vi "RAMP_close_single_scan_FPGA.vi"(0 "queue FPGA":refnum<queue>, 1 "queue ASI stage":refnum<queue>, 5 "queue CAMERA":refnum<queue>, 7 "Measure QPD":bool, 9 "queue piezo":refnum<queue>, 11 "error in":errorcluster, 12 "Z_position_file path":path, 14 "Illumination source":bool) -> (15 "error out":errorcluster)   [LabVIEW 2015]
uses:
  CONTROLS/Q_ASI_stage_element.ctl
  CONTROLS/Q_MCL_piezo_element.ctl
  CONTROLS/Q_camera_element.ctl
  CONTROLS/Q_FPGA_element.ctl
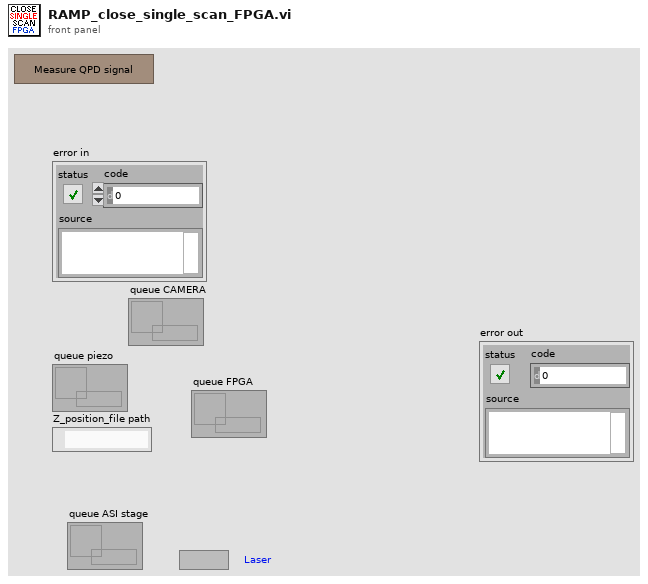
[diagram p1: front panel]
types:
  T1 = typedef "Q_FPGA_element.ctl" = cluster{"variant":variant, "Instruction":enum16{"FPGA_idle", "FPGA_initialize", "FPGA_error", "FPGA_security_stop", "FPGA_laser", "FPGA_start_stop_measure_QPD", "FPGA_measure_QPD", "FPGA_measure_QPD_noise", "FPGA_stop_measure_QPD", "FPGA_init_autofocus", "FPGA_init_single_scan", "FPGA_stop_single_scan", "FPGA_init_merFISH", "FPGA_measure_QPD_merFISH", "FPGA_init_scan_merFISH", "FPGA_scan_merFISH", "FPGA_close_merFISH", "FPGA_stop"}}
  T2 = typedef "Q_camera_element.ctl" = cluster{"variant":variant, "Instruction":enum16{"CAMERA_idle", "CAMERA_initialize", "CAMERA_error", "CAMERA_security_stop", "CAMERA_not_acquiring", "CAMERA_acquiring", "CAMERA_start_acquiring", "CAMERA_stop_acquiring", "CAMERA_change_exposure", "CAMERA_define_ROI", "CAMERA_cooler", "CAMERA_acquire_movie", "CAMERA_init_scan", "CAMERA_check_image_scan", "CAMERA_close_scan", "CAMERA_init_merFISH", "CAMERA_start_acquiring_merFISH", "CAMERA_close_scan_merFISH", "CAMERA_close_merFISH", "CAMERA_STOP"}}
  T3 = typedef "Q_MCL_piezo_element.ctl" = cluster{"variant":variant, "Instruction":enum16{"Piezo_idle", "Piezo_initialize", "Piezo_error", "Piezo_security_stop", "Piezo_read_z", "Piezo_move_z", "Piezo_keyboard_move", "Piezo_close_autofocus_calibration_ramp", "Piezo_change_init_state", "Piezo_init_autofocus", "Piezo_init_autofocus_merFISH_TL", "Piezo_autofocus", "Piezo_autofocus_merFISH_TL", "Piezo_stop_autofocus", "Piezo_stop_autofocus_merFISH_TL", "Piezo_autofocus_lost", "Piezo_resume_autofocus_merFISH_TL", "Piezo_check_z_position_merFISH_TL", "Piezo_init_ramp", "Piezo_move_z_ramp", "Piezo_close_ramp", "Piezo_close_merFISH", "Piezo_stop"}}
  T4 = typedef "Q_ASI_stage_element.ctl" = cluster{"variant":variant, "Instruction":enum16{"ASI_idle", "ASI_initialize", "ASI_error", "ASI_security_stop", "ASI_read_XYZ", "ASI_up", "ASI_down", "ASI_left", "ASI_right", "ASI_save_XY", "ASI_move_to_XY", "ASI_brightfield", "ASI_init_scan", "ASI_init_merFISH", "ASI_move_to_XY_merFISH", "ASI_move_to_Z_merFISH", "ASI_init_autofocus_search_merFISH", "ASI_close_autofocus_search_merFISH", "ASI_adjust_piezo_autofocus_merFISH", "ASI_set_piezo_autofocus_to_reference_position_merFISH_TL", "ASI_close_merFISH", "ASI_stop"}}
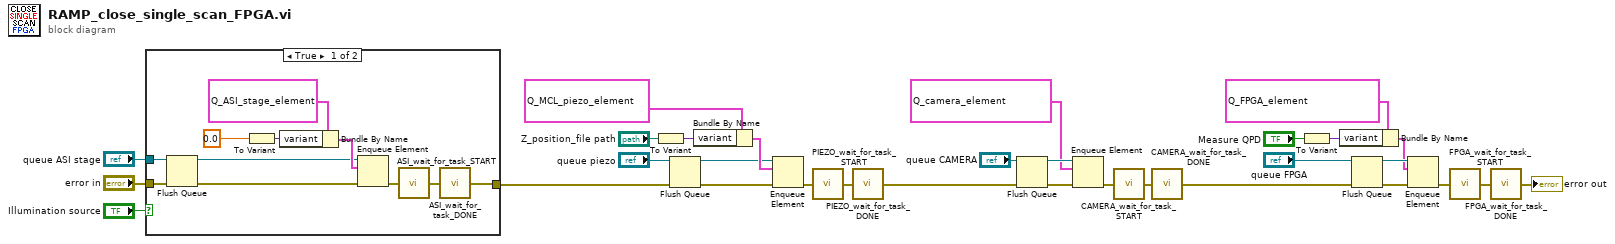
[diagram p0: block diagram]
diagram:
  n1 = case shown="True" "Illumination source" {
    tunnel: "error in" -> [w42 w43]
    tunnel: "queue ASI stage" -> [w41 _]
    tunnel: [w32 w43] -> w23
    frame True {
      n2 = Flush Queue(queue=w41, error in (no error)=w42) -> (queue out=w35:refnum<queue>, error out=w37:errorcluster)  [unwired: 1 out]
      n3 = To Variant(anything=0.0) -> (Variant=w39:variant)
      n4 = Bundle By Name(cluster=T4 {"variant"=variant, "Instruction"=enum."ASI_brightfield"} ("Q_ASI_stage"), "variant"=w39) -> (w36:T4)
      n5 = Enqueue Element(queue=w35, element=w36, error in (no error)=w37) -> (error out=w34:errorcluster)  [unwired: 1 in, 2 out]
      n6 = call "ASI_wait_for_task_START.vi"("error in"=w34) -> ("error out"=w33:errorcluster)
      n7 = call "ASI_wait_for_task_DONE.vi"("error in"=w33) -> ("error out"=w32:errorcluster)
    }
    frame False {
    }
  }
  n8 = To Variant(anything="Z_position_file path") -> (Variant=w22:variant)
  n9 = Flush Queue(queue="queue piezo", error in (no error)=w23) -> (queue out=w24:refnum<queue>, error out=w27:errorcluster)  [unwired: 1 out]
  n10 = Bundle By Name(cluster=T3 {"variant"=variant, "Instruction"=enum."Piezo_close_ramp"} ("Q_MCL_Piezo"), "variant"=w22) -> (w25:T3)
  n11 = Enqueue Element(queue=w24, element=w25, error in (no error)=w27) -> (error out=w20:errorcluster)  [unwired: 1 in, 2 out]
  n12 = call "PIEZO_wait_for_task_START.vi"("error in"=w20) -> ("error out"=w19:errorcluster)
  n13 = call "PIEZO_wait_for_task_DONE.vi"("error in"=w19) -> ("error out"=w14:errorcluster)
  n14 = Flush Queue(queue="queue CAMERA", error in (no error)=w14) -> (queue out=w16:refnum<queue>, error out=w15:errorcluster)  [unwired: 1 out]
  n15 = Enqueue Element(queue=w16, element=T2 {"variant"=variant, "Instruction"=enum."CAMERA_close_scan"} ("Q_ANDOR_element"), error in (no error)=w15) -> (error out=w17:errorcluster)  [unwired: 1 in, 2 out]
  n16 = call "CAMERA_wait_for_task_START.vi"("error in"=w17) -> ("error out"=w18:errorcluster)
  n17 = call "CAMERA_wait_for_task_DONE.vi"("error in"=w18) -> ("error out"=w11:errorcluster)
  n18 = To Variant(anything="Measure QPD") -> (Variant=w2:variant)
  n19 = Bundle By Name(cluster=T1 {"variant"=variant, "Instruction"=enum."FPGA_stop_single_scan"} ("element"), "variant"=w2) -> (w4:T1)
  n20 = Flush Queue(queue="queue FPGA", error in (no error)=w11) -> (queue out=w8:refnum<queue>, error out=w9:errorcluster)  [unwired: 1 out]
  n21 = Enqueue Element(queue=w8, element=w4, error in (no error)=w9) -> (error out=w7:errorcluster)  [unwired: 1 in, 2 out]
  n22 = call "FPGA_wait_for_task_START.vi"("error in"=w7) -> ("error out"=w6:errorcluster)
  n23 = call "FPGA_wait_for_task_DONE.vi"("error in"=w6) -> ("error out"=→"error out":errorcluster)
